vi "SPD.Strobe_Phase Sub Test.vi"(4 "Graph":refnum<vi>, 6 "Progress":refnum<vi>, 8 "Error In":errorcluster, 10 "SPD.Strobe_Phase Test Limits":T1, 11 "SPD.Stand Ctrl in":T2 {"spdDeviceSession"."hidSPD.Controller"."HV_bias" format="%#_6p, V"; "spdDeviceSession"."hidSPD.Controller"."TSet" format="%#_6p, DegC"}) -> (0 "Error Out":errorcluster, 1 "max phase":i32, 2 "max clicks":dbl, 3 "SPD.Stand Ctrl out":T2 {"spdDeviceSession"."hidSPD.Controller"."HV_bias" format="%#_6p, V"; "spdDeviceSession"."hidSPD.Controller"."TSet" format="%#_6p, DegC"})   [LabVIEW 2018]
uses:
  typedefs/SPD.Stand Ctrl.ctl
  Instruments/SPD HID Interface/hidSPDLibForLabView/LibVIs/hidSPD Controls/hidSPD Device Session.ctl
  Instruments/SPD HID Interface/hidSPDLibForLabView/LibVIs/hidSPD Controls/hidSPD Controller.ctl
  Instruments/KC705 DevBoard/typedefs/DevB.Session.ctl
  Instruments/KeySight 53230A/typedefs/FreqC.Session.ctl
  Instruments/KeySight 8164B/KeySight 8164B LAN InstrLib/typedefs/KeySight 8164B control.ctl
  Instruments/LeCroy SDA830/typedefs/LeCroy.Session.ctl
  typedefs/SPD.Events.ctl
  <vilib>/Utility/config.llb/Config Data RefNum.ctl
  typedefs/SPD.Meas Result.ctl
  SPD.Strobe_Phase Test Limits.ctl
  Instruments/SPD HID Interface/hidSPDLibForLabView/hidSPDLibForLabView.lvlib
  Instruments/KeySight 8164B/KeySight 8164B LAN InstrLib.lvlib
  <vilib>/Utility/config.llb/NI_LVConfig.lvlib
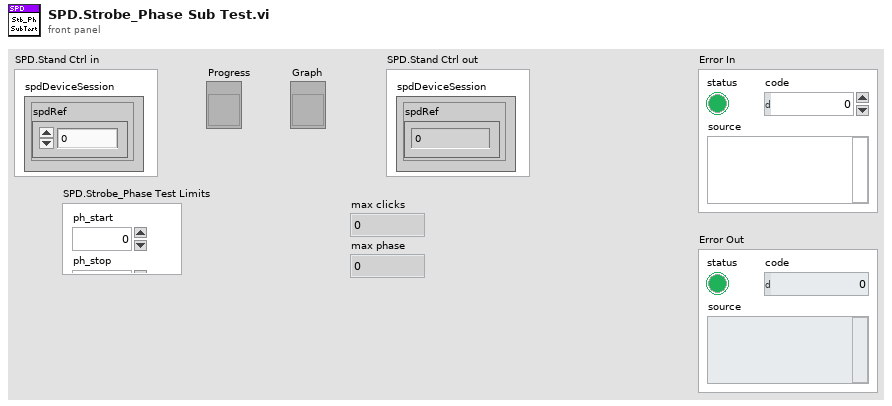
[diagram p1: front panel]
types:
  T1 = typedef "SPD.Strobe_Phase Test Limits.ctl" = cluster{"ph_start":i32, "ph_stop":i32, "ph_step":i32, "gate":dbl, "num of tests":dbl}
  T2 = typedef "SPD.Stand Ctrl.ctl" = cluster{"spdDeviceSession":T3, "DevBSession":T5, "FreqCSession":T6, "8164BSession":T7, "LeCroySession":T8, "Events":T9, "configFile":T10, "SPD.Result":T11}
  T3 = typedef "hidSPDLibForLabView.lvlib/hidSPD Device Session.ctl" = cluster{"spdRef":u64, "connected":bool, "spdName":string, "hidSPD.Controller":T4}
  T4 = typedef "hidSPDLibForLabView.lvlib/hidSPD Controller.ctl" = cluster{"TSet":sgl, "HV_bias":sgl, "DDS_stb_code":u16}
  T5 = typedef "DevB.Session.ctl" = cluster{"DevBRef":refnum<visa-resource-name>, "connected":bool}
  T6 = typedef "FreqC.Session.ctl" = cluster{"FreqCRef":refnum<visa-resource-name>, "timeout":dbl, "connected":bool}
  T7 = typedef "KeySight 8164B LAN InstrLib.lvlib/KeySight 8164B control.ctl" = cluster{"Connection ID":refnum<k5>, "Connected":bool, "Info":string, "Slots Info":string[]}
  T8 = typedef "LeCroy.Session.ctl" = cluster{"LeCroySession":refnum<visa-resource-name>, "connected":bool}
  T9 = typedef "SPD.Events.ctl" = cluster{"DCRTest":refnum<user-event>, "Stop":refnum<user-event>}
  T10 = typedef "NI_LVConfig.lvlib/Config Data RefNum.ctl" = refnum<k1>
  T11 = typedef "SPD.Meas Result.ctl" = cluster{"HV_Bias":dbl[], "Stb_code":dbl[], "Temprature":dbl[], "Data":dbl[][][][]}
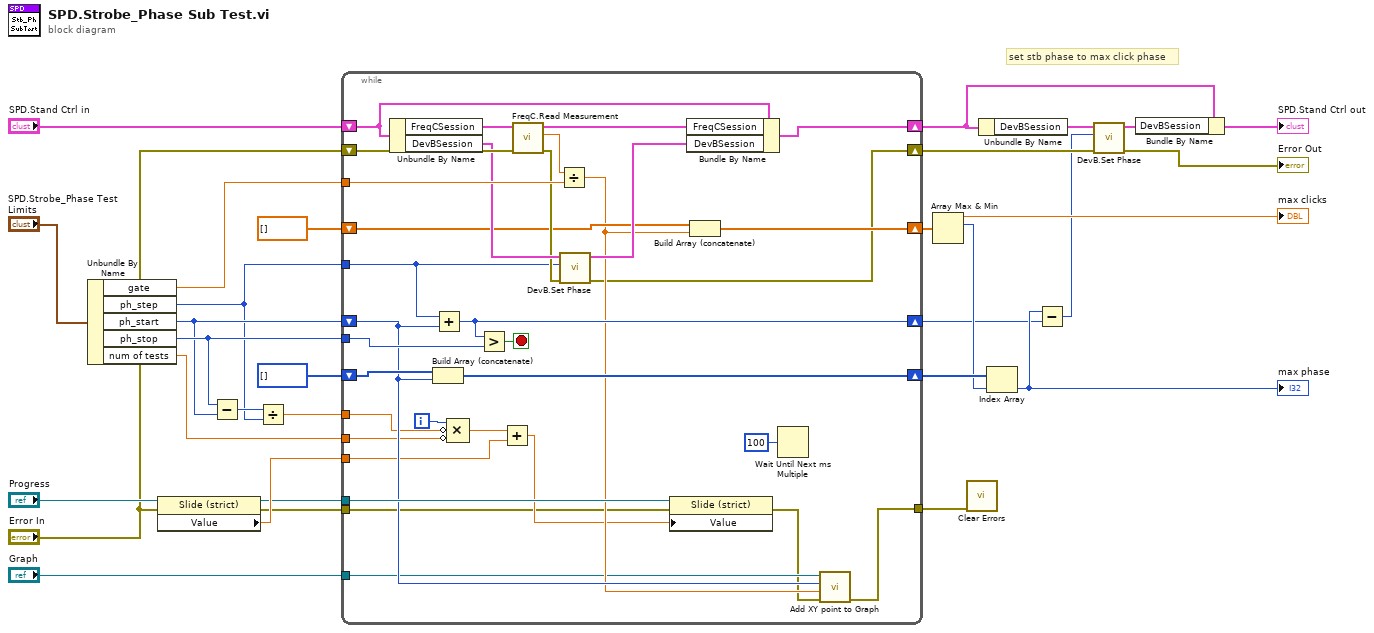
[diagram p0: block diagram]
diagram:
  # "set stb phase to max click phase"
  n1 = Unbundle By Name("SPD.Strobe_Phase Test Limits") -> ("gate"=w28:dbl, "ph_step"=w18:i32, "ph_start"=w19:i32, "ph_stop"=w20:i32, "num of tests"=w27:dbl)
  n2 = property class="Slide (strict)"(reference="Progress", error in="Error In") -> (reference out=w24:refnum<vi>, error out=w2:errorcluster, "Value"=w25:dbl)
  n3 = Subtract(x=w20, y=w19) -> (x-y=w21:i32)
  n4 = Divide(x=w21, y=w18) -> (x/y=w17:dbl)
  n5 = while {
    shift-right: [w35] -> w8
    shift-left: "Error In" -> [w60]
    shift-right: [w64] -> w10
    shift-left: "SPD.Stand Ctrl in" -> [w59]
    tunnel: w28 -> [w61]
    tunnel: w18 -> [w51]
    shift-right: [w52] -> w5
    shift-left: w19 -> [w43]
    tunnel: w20 -> [w54]
    tunnel: w27 -> [w37]
    shift-right: [w44] -> w16
    shift-left: dbl[] [] -> [w47]
    shift-right: [w45] -> w14
    shift-left: i32[] [] -> [w46]
    tunnel: w25 -> [w38]
    tunnel: w17 -> [w36]
    tunnel: "Graph" -> [w41]
    tunnel: w24 -> [w50]
    tunnel: w2 -> [w34]
    tunnel: [w33] -> w1
    i -> [w49]
    stop <- w53 stop-if-true
    n6 = Unbundle By Name(w59) -> ("FreqCSession"=w63:T6, "DevBSession"=w56:T5)
    n7 = Build Array (concatenate)(w46, w43) -> (w45:i32[])
    n8 = Add(x=w51, y=w43) -> (x+y=w52:i32)
    n9 = Compound Arithmetic op=MULTIPLY(w49, invert w36, invert w37) -> (w48:dbl)
    n10 = Greater?(x=w52, y=w54) -> (0:w53:bool)
    n11 = Add(x=w48, y=w38) -> (x+y=w39:dbl)
    n12 = call "FreqC.Read Measurement.vi"("error In"=w60, "FreqC Session in"=w63) -> ("error out"=w55:errorcluster, "Measurement"=w62:dbl, "FreqC Session out"=w58:T6)  [unwired: 7 in]
    n13 = Divide(x=w62, y=w61) -> (x/y=w42:dbl)
    n14 = call "DevB.Set Phase.vi"("error in (no error)"=w55, "Phase"=w51, "DevB Session in"=w56) -> ("error out"=w35:errorcluster, "DevB Session out"=w57:T5)  [unwired: 7 in]
    n15 = property class="Slide (strict)"(reference=w50, error in=w34, "Value"=w39) -> (error out=w40:errorcluster)  [unwired: 1 out]
    n16 = Bundle By Name(cluster=w59, "FreqCSession"=w58, "DevBSession"=w57) -> (w64:T2)
    n17 = Build Array (concatenate)(w47, w42) -> (w44:dbl[])
    n18 = Wait Until Next ms Multiple(millisecond multiple=u32 100) -> ()  [unwired: 1 out]
    n19 = call "Add XY point to Graph.vi"("error in (no error)"=w40, "Y"=w42, "X"=w43, "Graph in"=w41) -> ("error out"=w33:errorcluster)  [unwired: 6 in, 1 out]
  }
  n20 = Array Max & Min(array=w16) -> (max value=→"max clicks":dbl, max index (indices)=w13:i32)  [unwired: 2 out]
  n21 = call <vilib>:"Clear Errors.vi"("error in (no error)"=w1) -> ()  [unwired: 5 in, 2 out]
  n22 = Unbundle By Name(w10) -> ("DevBSession"=w12:T5)
  n23 = Index Array(array=w14, index=w13) -> (element=w6:i32)
  "max phase" <- w6
  n24 = Subtract(x=w6, y=w5) -> (x-y=w4:i32)
  n25 = call "DevB.Set Phase.vi"("error in (no error)"=w8, "Phase"=w4, "DevB Session in"=w12) -> ("error out"=→"Error Out":errorcluster, "DevB Session out"=w11:T5)  [unwired: 7 in]
  n26 = Bundle By Name(cluster=w10, "DevBSession"=w11) -> (→"SPD.Stand Ctrl out":T2)
